vi "Move to poin - polart.vi"(7 "Speed":dbl, 11 "Input string":string) -> ()   [LabVIEW 2011]
uses:
  <vilib>/addons/control/pid/pid.llb/PID (DBL).vi
  <vilib>/regexp/Match Regular Expression.xnode
  <vilib>/addons/control/pid/NI_PID_pid.lvlib
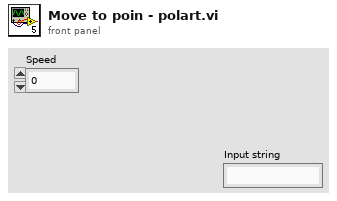
[diagram p1: front panel]
types:
  T1 = typedef "WPI_EncoderDevRef.ctl" = cluster{"DevStatus":errorcluster, "EncoderIndex":T2, "CounterIndex":T3, "DistancePerCount":dbl, "Decoding Type":T4}
  T2 = typedef "FPGA_EncoderIdx.ctl" = enum8{"Enc 0", "Enc 1", "Enc 2", "Enc 3", "Invalid"}
  T3 = typedef "FPGA_CounterCtrSystemIndex.ctl" = enum8{"Ctr 0", "Ctr 1", "Ctr 2", "Ctr 3", "Ctr 4", "Ctr 5", "Ctr 6", "Ctr 7", "Invalid"}
  T4 = typedef "WPI_EncoderType.ctl" = enum16{"1x", "2x", "4x"}
  T5 = typedef "WPI_MotorControlDeviceRef.ctl" = cluster{"DeviceStatus":errorcluster, "Type":enum16{"PWM", "CAN"}, "PWM":cluster{"Digital Module":T6, "PWM Channel":T7, "DeadBand":T8}, "CAN":cluster{"Device Number":u8, "Control Mode":T9, "Semaphore":T10, "Max Vout":dbl}, "Invert":bool, "TransformRef":T11, "InvTransformRef":T11}
  T6 = typedef "FPGA_TypedefDigitalModule.ctl" = enum16{"Digital Module 1", "Digital Module 2"}
  T7 = typedef "FPGA_DIOPWMChannel.ctl" = enum8{"PWM 1", "PWM 2", "PWM 3", "PWM 4", "PWM 5", "PWM 6", "PWM 7", "PWM 8", "PWM 9", "PWM 10", "Invalid"}
  T8 = typedef "WPI_PWMDeadband.ctl" = cluster{"Name":string, "maxPositivePwm":i32, "minPositivePwm":i32, "centerPwm":i32, "maxNegativePwm":i32, "minNegativePwm":i32, "angularRange":u16}
  T9 = typedef "WPI_CANJaguar_ControlMode.ctl" = enum8{"Percent VBus", "Current", "Speed", "Position", "Voltage"}
  T10 = typedef "Semaphore RefNum" = refnum<k1>
  T11 = typedef "WPI_PWMTransform_ConPane.ctl" = refnum<vi>
  T12 = cluster{"proportional gain (Kc)":dbl, "integral time (Ti, min)":dbl, "derivative time (Td, min)":dbl}
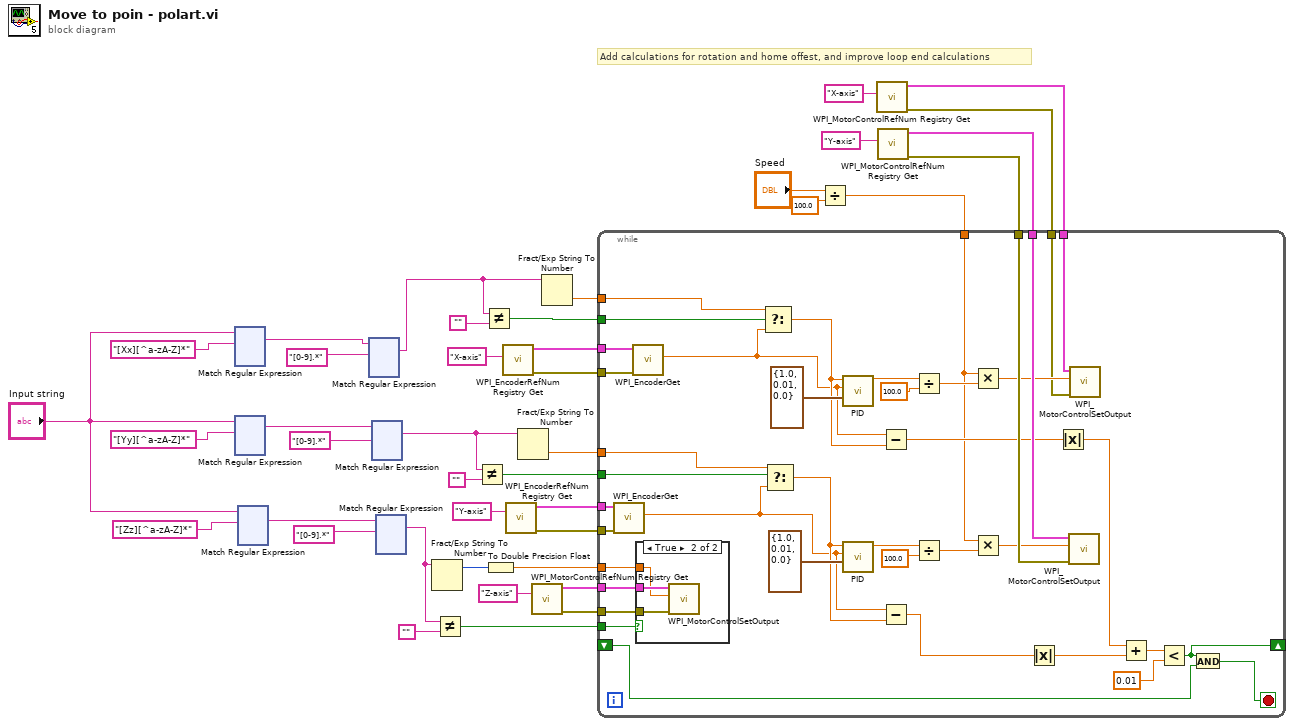
[diagram p0: block diagram]
diagram:
  # "Add calculations for rotation and home offest, and improve loop end calculations"
  n1 = xnode "Match Regular Expression"("input string"="Input string", "regular expression"="[Xx][^a-zA-Z]*") -> ("whole match"=w36:string)  [unwired: 4 in, 4 out]
  n2 = xnode "Match Regular Expression"("input string"="Input string", "regular expression"="[Yy][^a-zA-Z]*") -> ("whole match"=w32:string)  [unwired: 4 in, 4 out]
  n3 = xnode "Match Regular Expression"("input string"="Input string", "regular expression"="[Zz][^a-zA-Z]*") -> ("whole match"=w33:string)  [unwired: 4 in, 4 out]
  n4 = xnode "Match Regular Expression"("input string"=w36, "regular expression"="[0-9].*") -> ("whole match"=w10:string)  [unwired: 4 in, 4 out]
  n5 = xnode "Match Regular Expression"("input string"=w32, "regular expression"="[0-9].*") -> ("whole match"=w8:string)  [unwired: 4 in, 4 out]
  n6 = xnode "Match Regular Expression"("input string"=w33, "regular expression"="[0-9].*") -> ("whole match"=w6:string)  [unwired: 4 in, 4 out]
  n7 = Fract/Exp String To Number(string=w6) -> (offset past number=w14:i32)  [unwired: 3 in, 1 out]
  n8 = Not Equal?(x=w6, y="") -> (x != y?=w4:bool)
  n9 = Not Equal?(x=w8, y="") -> (x != y?=w7:bool)
  n10 = Not Equal?(x=w10, y="") -> (x != y?=w12:bool)
  n11 = To Double Precision Float(number=w14) -> (double precision float=w13:dbl)
  n12 = call <vilib>:"WPI_EncoderRefNum Registry Get.vi"("refnum name"="X-axis") -> ("error out"=w27:errorcluster, "EncoderDevRef"=w26:T1)  [unwired: 9 in]
  n13 = call <vilib>:"WPI_EncoderRefNum Registry Get.vi"("refnum name"="Y-axis") -> ("error out"=w23:errorcluster, "EncoderDevRef"=w24:T1)  [unwired: 9 in]
  n14 = Fract/Exp String To Number(string=w8) -> (number=w25:dbl)  [unwired: 3 in, 1 out]
  n15 = call <vilib>:"WPI_MotorControlRefNum Registry Get.vi"("refnum name"="Z-axis") -> ("error out"=w15:errorcluster, "MotorControlDevRef"=w16:T5)  [unwired: 9 in]
  n16 = Fract/Exp String To Number(string=w10) -> (number=w28:dbl)  [unwired: 3 in, 1 out]
  n17 = Divide(x="Speed", y=100.0) -> (x/y=w1:dbl)
  n18 = call <vilib>:"WPI_MotorControlRefNum Registry Get.vi"("refnum name"="X-axis") -> ("error out"=w20:errorcluster, "MotorControlDevRef"=w21:T5)  [unwired: 9 in]
  n19 = call <vilib>:"WPI_MotorControlRefNum Registry Get.vi"("refnum name"="Y-axis") -> ("error out"=w17:errorcluster, "MotorControlDevRef"=w18:T5)  [unwired: 9 in]
  n20 = while {
    tunnel: w28 -> [w59]
    tunnel: w27 -> [w79]
    tunnel: w26 -> [w78]
    tunnel: w25 -> [w51]
    tunnel: w24 -> [w75]
    tunnel: w23 -> [w74]
    shift-right: [w68] -> _
    shift-left: _ -> [w67]
    tunnel: w21 -> [w66]
    tunnel: w20 -> [w45]
    tunnel: w18 -> [w65]
    tunnel: w17 -> [w64]
    tunnel: w16 -> [w63]
    tunnel: w15 -> [w62]
    tunnel: w13 -> [w61]
    tunnel: w12 -> [w58]
    tunnel: w7 -> [w53]
    tunnel: w4 -> [w49]
    tunnel: w1 -> [w42]
    stop <- w48 stop-if-true
    n21 = call <vilib>:"WPI_EncoderGet.vi"("error in (no error)"=w74, "EncoderDevRef"=w75) -> ("Distance"=w50:dbl)  [unwired: 4 in, 5 out]
    n22 = call <vilib>:"WPI_EncoderGet.vi"("error in (no error)"=w79, "EncoderDevRef"=w78) -> ("Distance"=w57:dbl)  [unwired: 4 in, 5 out]
    n23 = case shown="True" w49 {
      tunnel: w63 -> [_ w84]
      tunnel: w62 -> [_ w83]
      tunnel: w61 -> [_ w82]
      frame False {
      }
      frame True {
        n24 = call <vilib>:"WPI_MotorControlSetOutput.vi"("error in (no error)"=w83, "Output"=w82, "MotorControlDevRef"=w84) -> ()  [unwired: 7 in, 2 out]
      }
    }
    n25 = Select(t=w59, s=w58, f=w57) -> (s? t:f=w60:dbl)
    n26 = Select(t=w51, s=w53, f=w50) -> (s? t:f=w52:dbl)
    n27 = call-poly <vilib>:"PID.vi"("PID gains"=T12 {"proportional gain (Kc)"=1.0, "integral time (Ti, min)"=0.01, "derivative time (Td, min)"=0.0}, "process variable"=w57, "setpoint"=w60) -> ("output"=w72:dbl)  [unwired: 7 in, 1 out]
    n28 = call-poly <vilib>:"PID.vi"("PID gains"=T12 {"proportional gain (Kc)"=1.0, "integral time (Ti, min)"=0.01, "derivative time (Td, min)"=0.0}, "process variable"=w50, "setpoint"=w52) -> ("output"=w73:dbl)  [unwired: 7 in, 1 out]
    n29 = Subtract(x=w57, y=w60) -> (x-y=w55:dbl)
    n30 = Subtract(x=w50, y=w52) -> (x-y=w71:dbl)
    n31 = Divide(x=w72, y=100.0) -> (x/y=w46:dbl)
    n32 = Divide(x=w73, y=100.0) -> (x/y=w43:dbl)
    n33 = Multiply(x=w42, y=w46) -> (x*y=w47:dbl)
    n34 = Multiply(x=w42, y=w43) -> (x*y=w44:dbl)
    n35 = Absolute Value(x=w71) -> (abs(x)=w56:dbl)
    n36 = Absolute Value(x=w55) -> (abs(x)=w54:dbl)
    n37 = call <vilib>:"WPI_MotorControlSetOutput.vi"("error in (no error)"=w64, "Output"=w44, "MotorControlDevRef"=w65) -> ()  [unwired: 7 in, 2 out]
    n38 = call <vilib>:"WPI_MotorControlSetOutput.vi"("error in (no error)"=w45, "Output"=w47, "MotorControlDevRef"=w66) -> ()  [unwired: 7 in, 2 out]
    n39 = Add(x=w54, y=w56) -> (x+y=w70:dbl)
    n40 = Less?(x=w70, y=0.01) -> (x < y?=w68:bool)
    n41 = And(x=w68, y=w67) -> (x .and. y?=w48:bool)
  }
